vi "Access Module Ranges.vi"(8 "error in":errorcluster, 11 "3300 in":refnum<class "3300.lvclass">) -> (0 "error out":errorcluster, 2 "Ranges":cluster{"Low":dbl, "High":dbl}[](array[cluster]), 3 "3300 out":refnum<class "3300.lvclass">)   [LabVIEW 2019, in "3300.lvlib" / "3300.lvclass"]
uses:
  Library/3300.lvclass
  C:/Users/Public/Documents/Development/builds/Instruments/Electronic Load.lvlibp/Library/Electronic Load.lvclass
  builds/Instruments/Electronic Load.lvlibp/Accessors/Trigger/Read Pulse Mode.vi
  Accessors/Read Active Module.vi
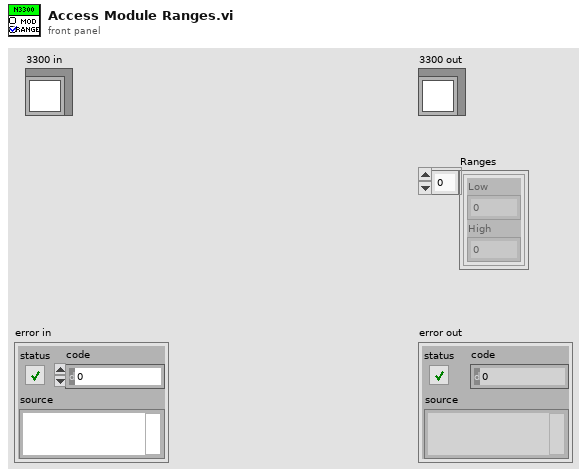
[diagram p1: front panel]
types:
  T1 = typedef "Electronic Load.lvlibp/Electronic Load.lvclass/E-Load Mode.ctl" = enum16{"Current", "Resistance", "Voltage"}
  T2 = typedef "3300.lvlib/3300.lvclass/Modules.ctl" = enum16{"N3302A", "N3303A", "N3304A", "N3305A", "N3306A", "N3307A"}
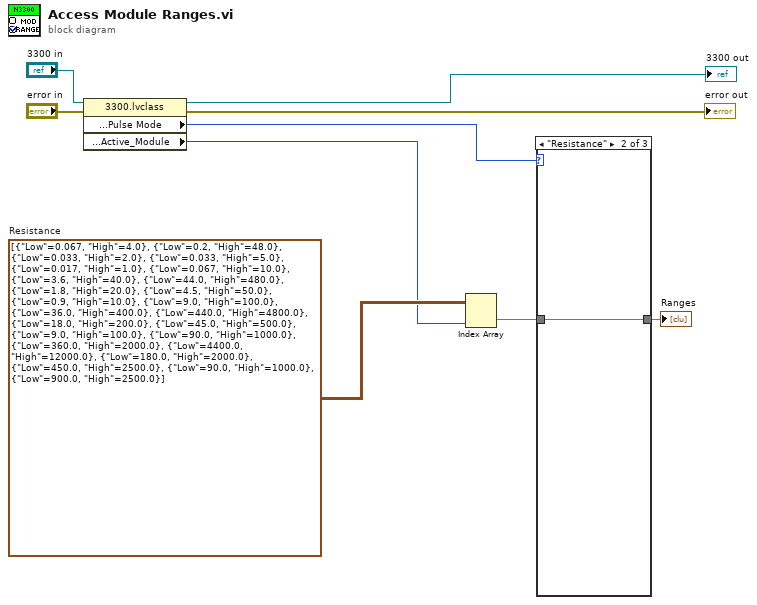
[diagram p0: block diagram]
diagram:
  w4 = cluster{"Low":dbl, "High":dbl}[][] [[{"Low"=0.067, "High"=4.0}, {"Low"=0.2, "High"=48.0}, {"Low"=0.033, "High"=2.0}, {"Low"=0.033, "High"=5.0}, {"Low"=0.017, "High"=1.0}, {"Low"=0.067, "High"=10.0}], [{"Low"=3.6, "High"=40.0}, {"Low"=44.0, "High"=480.0}, {"Low"=1.8, "High"=20.0}, {"Low"=4.5, "High"=50.0}, {"Low"=0.9, "High"=10.0}, {"Low"=9.0, "High"=100.0}], [{"Low"=36.0, "High"=400.0}, {"Low"=440.0, "High"=4800.0}, {"Low"=18.0, "High"=200.0}, {"Low"=45.0, "High"=500.0}, {"Low"=9.0, "High"=100.0}, {"Low"=90.0, "High"=1000.0}], [{"Low"=360.0, "High"=2000.0}, {"Low"=4400.0, "High"=12000.0}, {"Low"=180.0, "High"=2000.0}, {"Low"=450.0, "High"=2500.0}, {"Low"=90.0, "High"=1000.0}, {"Low"=900.0, "High"=2500.0}]]  # Resistance
  n1 = property class="3300.lvclass"(reference="3300 in", error in="error in") -> (reference out=→"3300 out":refnum<class "3300.lvclass">, error out=→"error out":errorcluster, "Accessors:Settings:Pulse:Pulse Mode"=w1:T1, "Private:Accessors:Active_Module"=w2:T2)
  n2 = Index Array(array=w4, index (col)=w2) -> (element=w5:cluster{"Low":dbl, "High":dbl}[])  [unwired: 1 in]
  n3 = case shown="\"Resistance\"" w1 {
    tunnel: w5 -> [_ w10 _]
    tunnel: [_ w10 _] -> w3
    frame "Current", Default {
    }
    frame "Resistance" {
    }
    frame "Voltage" {
    }
  }
  "Ranges" <- w3
